vi "Initial Values-format and values-DBL.vi"() -> (1 "Values Array":dbl[](array[numeric]), 3 "Keys Array":T1)   [LabVIEW 2013]
uses:
  Typedefs/Ini file interface (DBL).ctl
  User Interface/Visualisation/Functional Imaging Viewer/Typedefs/Get-Set-Clear Control.ctl
  Global Variables/gl_UI Ctrl Refs.vi
  User Interface/Visualisation/Timelapse Viewer/Globals/gl_Time series viewer globals.vi
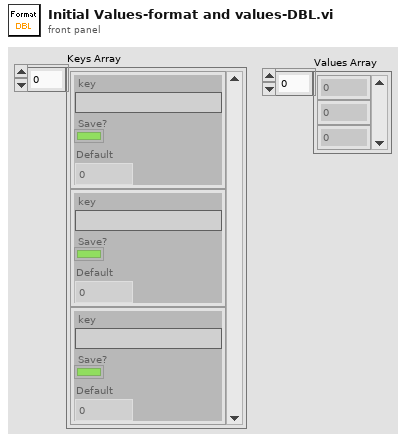
[diagram p1: front panel]
types:
  T1 = typedef "Ini file interface (DBL).ctl" = cluster{"key":string, "Save?":bool, "Default":dbl}[]
  T2 = typedef "Get-Set-Clear Control.ctl" = enum16{"Get", "Set", "Clear"}
  T3 = typedef "UI ctrl refs cluster.ctl" = cluster{"Top level VI path":path, "Top level VI ref":refnum<vi>, "User menu ref":refnum<k9>, "Sub Panel control":refnum<vi>, "Imaging Param Tab":refnum<vi>, "Occurrence-Start drivers":refnum<k4>, "Occurrence-Speed logging initialised":refnum<k4>, "Occurrence-XYZ stage initialised":refnum<k4>, "Exit button":refnum<vi>, "Status ind":refnum<vi>, "Return to Origin":refnum<vi>, "Speed Logging":refnum<vi>, "Time Lapse":refnum<vi>, "Live Imaging":refnum<vi>, "AOL Z Stack":refnum<vi>, "Motor Z Stack":refnum<vi>, "Funct Acq button":refnum<vi>, "Hard Shutter":refnum<vi>, "Virtual Shutter":refnum<vi>, "Laser Power":refnum<vi>, "AOL Mode":refnum<vi>, "Frame Size":refnum<vi>, "Field of View":refnum<vi>, "Dwell Time":refnum<vi>, "Zoom":refnum<vi>, "AOL Z":refnum<vi>, "Objective":refnum<vi>, "Axis":refnum<vi>, "Paths & Names":refnum<vi>, "Experiment folder path (ind.)":refnum<vi>, "Last State (Ind.)":refnum<vi>, "Laser wavelength ind (nm)":refnum<vi>, "Averages":refnum<vi>, "Angle (degrees)":refnum<vi>, "X centre":refnum<vi>, "Y centre":refnum<vi>, "Plane Mode":refnum<vi>, "# Planes":refnum<vi>, "Z Start":refnum<vi>, "Z Stop":refnum<vi>, "Z Step":refnum<vi>, "PMT 1":refnum<vi>, "PMT 2":refnum<vi>, "Stage XYZ Position":refnum<vi>, "Pockels@Z Start":refnum<vi>, "Pockels@Z Stop":refnum<vi>, "Obtain Z Start":refnum<vi>, "Obtain Z Stop":refnum<vi>, "Live stim.trig.period":refnum<vi>, "Live stim.trig.enable":refnum<vi>, "Funct. Acq. Pockels Modulation":refnum<vi>, "Enable Video Recording":refnum<vi>, "Video Record-Live Imaging":refnum<vi>, "Video Record-Funct acq":refnum<vi>, "AOL Z-stack Chirps Ready (ind)":refnum<vi>, "Center freq ind (nm)":refnum<vi>, "Logging queue (ind)":refnum<vi>, "Back aperture power (ind.)":refnum<vi>, "Power after objective (ind.)":refnum<vi>, "Switch user":refnum<vi>}
  T4 = typedef "AOL_Globals.ctl" = cluster{"Imaging Protocol":T5, "Number of POI":u16, "Number of Miniscans":u16, "Number of Trials":u16, "Number of Cycles ":u64, "# Averaged Frames":u16, "Laser power (%)":u8, "Pockels":dbl, "Acquisition Length (sec)":dbl, "Fill time (us)":dbl, "POI Dwell time (us)":dbl, "Miniscan Dwell time per pixel (us)":dbl, "PMT 1":dbl, "PMT 2":dbl, "Back Apperture":dbl, "Frame Size":T6, "Center Frequency":dbl, "Field of View":dbl, "DwellTime (us)":dbl, "Wavelength (nm)":dbl, "Zoom":dbl, "AOL Z":dbl, "AOL Mode":T7, "GridXY":dbl, "GridZ":dbl, "TriggerPeriod (sec)":dbl, "Number of Pixels in Miniscan":u16, "Experiment folder path":path, "X centre":dbl, "Y centre":dbl, "Angle (degrees)":dbl, "Plane Mode":T8, "Threshold":u16[], "Regenerate Chirps":bool, "Rectangle ROI length (pixels)":u16, "Rectangle ROI height (pixels)":u16, "AOD fill":u16, "Samples Wait after Trigger":u16, "StartUp Delay":i32, "Slip Cycle":u32, "Add Cycle":bool}
  T5 = typedef "Imaging Protocols enum.ctl" = enum16{"AOL Z-Stack", "Motor Z Stack", "Functional Acquisition", "Single Plane Acquisition", "Volume Acquisition", "Live Imaging", "Live Plane Imaging", "Live Volume Imaging"}
  T6 = typedef "Frame Size.ctl" = u16
  T7 = typedef "AOL modes.ctl" = enum16{"Raster", "Structural", "Pointing", "Mini Scan", "Alignment"}
  T8 = typedef "Plane Mode.ctl" = u16
  T9 = typedef "Stitch layout spec cluster.ctl" = cluster{"Timelapse image":cluster{"Image position":T10}, "Cam 1":cluster{"Image position":T10}, "Cam 2":cluster{"Image position":T10}, "Cam 3":cluster{"Image position":T10}, "Cam 4":cluster{"Image position":T10}}
  T10 = typedef "Image stitching positions.ctl" = enum16{"Top left", "Top right", "Bottom left", "Bottom right", "Not used"}
  T11 = typedef "PMT control knob.ctl" = u16
  T12 = typedef "Custom slider-horisontal.ctl" = cluster{dbl, dbl}
  T13 = typedef "Speed graph behaviour enum.ctl" = enum16{"Scrolling data", "Scrolling cursor"}
  T14 = typedef "AVI implementation enum.ctl" = enum16{"AVI1", "AVI2"}
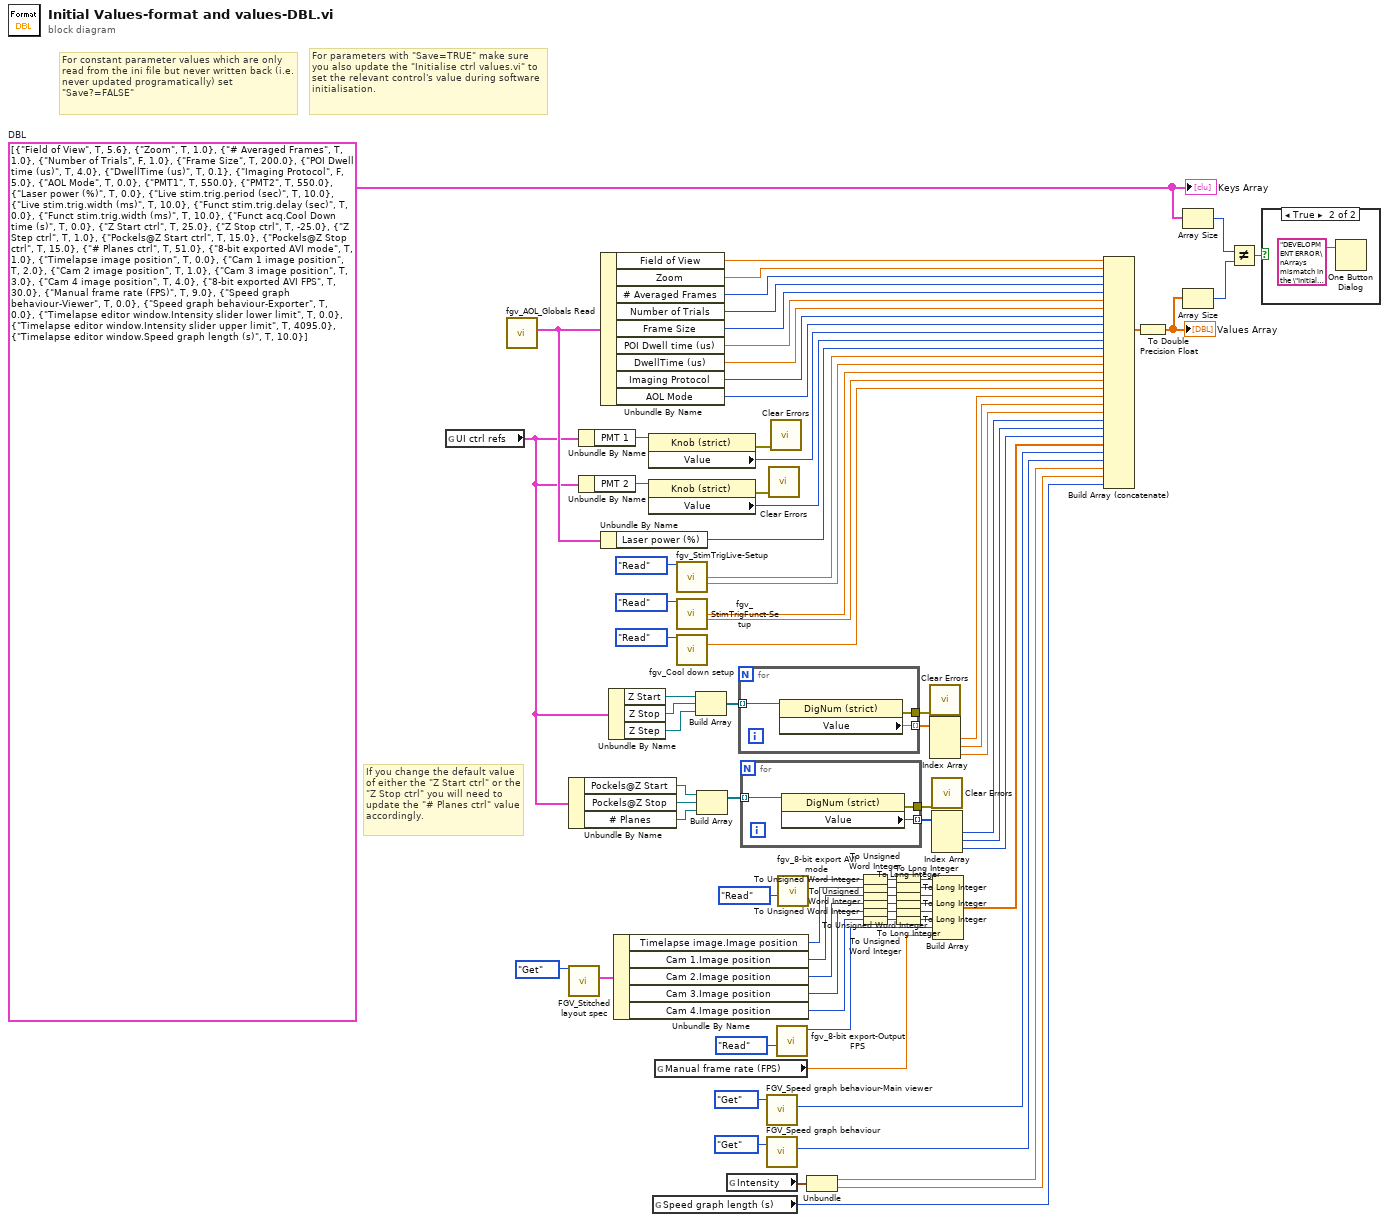
[diagram p0: block diagram]
diagram:
  w56 = T1 [{"key"="Field of View", "Save?"=TRUE, "Default"=5.6}, {"key"="Zoom", "Save?"=TRUE, "Default"=1.0}, {"key"="# Averaged Frames", "Save?"=TRUE, "Default"=1.0}, {"key"="Number of Trials", "Save?"=FALSE, "Default"=1.0}, {"key"="Frame Size", "Save?"=TRUE, "Default"=200.0}, {"key"="POI Dwell time (us)", "Save?"=TRUE, "Default"=4.0}, {"key"="DwellTime (us)", "Save?"=TRUE, "Default"=0.1}, {"key"="Imaging Protocol", "Save?"=FALSE, "Default"=5.0}, {"key"="AOL Mode", "Save?"=TRUE, "Default"=0.0}, {"key"="PMT1", "Save?"=TRUE, "Default"=550.0}, {"key"="PMT2", "Save?"=TRUE, "Default"=550.0}, {"key"="Laser power (%)", "Save?"=TRUE, "Default"=0.0}, {"key"="Live stim.trig.period (sec)", "Save?"=TRUE, "Default"=10.0}, {"key"="Live stim.trig.width (ms)", "Save?"=TRUE, "Default"=10.0}, {"key"="Funct stim.trig.delay (sec)", "Save?"=TRUE, "Default"=0.0}, {"key"="Funct stim.trig.width (ms)", "Save?"=TRUE, "Default"=10.0}, {"key"="Funct acq.Cool Down time (s)", "Save?"=TRUE, "Default"=0.0}, {"key"="Z Start ctrl", "Save?"=TRUE, "Default"=25.0}, {"key"="Z Stop ctrl", "Save?"=TRUE, "Default"=-25.0}, {"key"="Z Step ctrl", "Save?"=TRUE, "Default"=1.0}, {"key"="Pockels@Z Start ctrl", "Save?"=TRUE, "Default"=15.0}, {"key"="Pockels@Z Stop ctrl", "Save?"=TRUE, "Default"=15.0}, {"key"="# Planes ctrl", "Save?"=TRUE, "Default"=51.0}, {"key"="8-bit exported AVI mode", "Save?"=TRUE, "Default"=1.0}, {"key"="Timelapse image position", "Save?"=TRUE, "Default"=0.0}, {"key"="Cam 1 image position", "Save?"=TRUE, "Default"=2.0}, {"key"="Cam 2 image position", "Save?"=TRUE, "Default"=1.0}, {"key"="Cam 3 image position", "Save?"=TRUE, "Default"=3.0}, {"key"="Cam 4 image position", "Save?"=TRUE, "Default"=4.0}, {"key"="8-bit exported AVI FPS", "Save?"=TRUE, "Default"=30.0}, {"key"="Manual frame rate (FPS)", "Save?"=TRUE, "Default"=9.0}, {"key"="Speed graph behaviour-Viewer", "Save?"=TRUE, "Default"=0.0}, {"key"="Speed graph behaviour-Exporter", "Save?"=TRUE, "Default"=0.0}, {"key"="Timelapse editor window.Intensity slider lower limit", "Save?"=TRUE, "Default"=0.0}, {"key"="Timelapse editor window.Intensity slider upper limit", "Save?"=TRUE, "Default"=4095.0}, {"key"="Timelapse editor window.Speed graph length (s)", "Save?"=TRUE, "Default"=10.0}]  # DBL
  # "If you change the default value of either the \"Z Start ctrl\" or the \"Z Stop ctrl\" you will need to update the \"# Planes ctrl\" value accordingly."
  # "For parameters with \"Save=TRUE\" make sure you also update the \"Initialise ctrl values.vi\" to set the relevant control's value during software initialisation."
  # "For constant parameter values which are only read from the ini file but never written back (i.e. never updated programatically) set \"Save?=FALSE\""
  n1 = global read "gl_UI Ctrl Refs.vi" "UI ctrl refs"() -> (w45:T3)
  n2 = call "fgv_AOL_Globals Read.vi"() -> ("AOL_Globals"=w70:T4)  [unwired: 9 in, 2 out]
  n3 = Unbundle By Name(w45) -> ("Pockels@Z Start"=w46:refnum<vi>, "Pockels@Z Stop"=w47:refnum<vi>, "# Planes"=w37:refnum<vi>)
  n4 = call "FGV_Stitched layout spec.vi"("Function"=Get-Set-Clear_Control."Get") -> ("Stitch layout spec"=w31:T9)  [unwired: 9 in, 1 out]
  n5 = Unbundle By Name(w45) -> ("PMT 1"=w73:refnum<vi>)
  n6 = Unbundle By Name(w45) -> ("PMT 2"=w72:refnum<vi>)
  n7 = Unbundle By Name(w70) -> ("Field of View"=w59:dbl, "Zoom"=w60:dbl, "# Averaged Frames"=w62:u16, "Number of Trials"=w61:u16, "Frame Size"=w63:T6, "POI Dwell time (us)"=w64:dbl, "DwellTime (us)"=w65:dbl, "Imaging Protocol"=w66:T5, "AOL Mode"=w67:T7)
  n8 = Unbundle By Name(w70) -> ("Laser power (%)"=w71:u8)
  n9 = Unbundle By Name(w45) -> ("Z Start"=w52:refnum<vi>, "Z Stop"=w50:refnum<vi>, "Z Step"=w49:refnum<vi>)
  n10 = Unbundle By Name(w31) -> ("Timelapse image.Image position"=w30:T10, "Cam 1.Image position"=w29:T10, "Cam 2.Image position"=w28:T10, "Cam 3.Image position"=w27:T10, "Cam 4.Image position"=w26:T10)
  n11 = property class="Knob (strict)"(reference=w73) -> (error out=w74:errorcluster, "Value"=w68:T11)  [unwired: 1 in, 1 out]
  n12 = property class="Knob (strict)"(reference=w72) -> (error out=w75:errorcluster, "Value"=w69:T11)  [unwired: 1 in, 1 out]
  n13 = global read "gl_Time series viewer globals.vi" "Speed graph length (s)"() -> (w1:i32)
  n14 = global read "gl_Time series viewer globals.vi" "Manual frame rate (FPS)"() -> (w12:dbl)
  n15 = call "fgv_StimTrigLive-Setup.vi"("Function"=enum16{"Intialize", "Write", "Read", "Clear"}."Read") -> ("Live stim.trig.period (sec)"=w78:dbl, "Live stim.trig.width (ms)"=w79:dbl)  [unwired: 11 in, 2 out]
  n16 = call "fgv_StimTrigFunct-Setup.vi"("Function"=enum16{"Intialize", "Write", "Read", "Clear"}."Read") -> ("Funct stim.trig.delay (sec)"=w80:dbl, "Funct stim.trig.width (ms)"=w81:dbl)  [unwired: 11 in, 2 out]
  n17 = call "fgv_Cool down setup.vi"("Function"=enum16{"Intialize", "Write", "Read", "Clear"}."Read") -> ("Cool-down time (s)"=w83:dbl)  [unwired: 12 in, 2 out]
  n18 = Build Array(w52, w50, w49) -> (w51:refnum<vi>[])
  n19 = Build Array(w46, w47, w37) -> (w43:refnum<vi>[])
  n20 = global read "gl_Time series viewer globals.vi" "Intensity"() -> (w4:T12)
  n21 = for {
    tunnel: w51 -> [w86] mode=indexing
    tunnel: [w85] -> w48 mode=indexing
    tunnel: [w84] -> w10
    n22 = property class="DigNum (strict)"(reference=w86) -> (error out=w84:errorcluster, "Value"=w85:dbl)  [unwired: 1 in, 1 out]
  }
  n23 = for {
    tunnel: w43 -> [w89] mode=indexing
    tunnel: [w88] -> w44 mode=indexing
    tunnel: [w87] -> w9
    n24 = property class="DigNum (strict)"(reference=w89) -> (error out=w87:errorcluster, "Value"=w88:u16)  [unwired: 1 in, 1 out]
  }
  n25 = call "FGV_Speed graph behaviour-Main viewer.vi"("Function"=Get-Set-Clear_Control."Get") -> ("Speed graph behaviour"=w6:T13)  [unwired: 9 in, 1 out]
  n26 = call "FGV_Speed graph behaviour.vi"("Function"=Get-Set-Clear_Control."Get") -> ("Speed graph behaviour"=w5:T13)  [unwired: 9 in, 1 out]
  n27 = call <vilib>:"Clear Errors.vi"("error in (no error)"=w75) -> ()  [unwired: 6 in, 1 out]
  n28 = call <vilib>:"Clear Errors.vi"("error in (no error)"=w74) -> ()  [unwired: 6 in, 1 out]
  n29 = call "fgv_8-bit export-Output FPS.vi"("Function"=enum16{"Intialize", "Write", "Read", "Clear"}."Read") -> ("Frames Per Second"=w35:u32)  [unwired: 9 in, 1 out]
  n30 = call "fgv_8-bit export AVI mode.vi"("Function"=enum16{"Intialize", "Write", "Read", "Clear"}."Read") -> ("AVI mode"=w33:T14)  [unwired: 9 in, 1 out]
  n31 = Unbundle(w4) -> (w3:dbl, w2:dbl)
  n32 = To Unsigned Word Integer(number=w33) -> (unsigned 16bit integer=w19:u16)
  n33 = To Unsigned Word Integer(number=w30) -> (unsigned 16bit integer=w18:u16)
  n34 = To Unsigned Word Integer(number=w29) -> (unsigned 16bit integer=w17:u16)
  n35 = To Unsigned Word Integer(number=w28) -> (unsigned 16bit integer=w16:u16)
  n36 = To Unsigned Word Integer(number=w27) -> (unsigned 16bit integer=w15:u16)
  n37 = To Unsigned Word Integer(number=w26) -> (unsigned 16bit integer=w14:u16)
  n38 = To Long Integer(number=w19) -> (32bit integer=w24:i32)
  n39 = To Long Integer(number=w18) -> (32bit integer=w25:i32)
  n40 = To Long Integer(number=w17) -> (32bit integer=w23:i32)
  n41 = To Long Integer(number=w16) -> (32bit integer=w22:i32)
  n42 = To Long Integer(number=w15) -> (32bit integer=w21:i32)
  n43 = To Long Integer(number=w14) -> (32bit integer=w20:i32)
  n44 = call <vilib>:"Clear Errors.vi"("error in (no error)"=w10) -> ()  [unwired: 6 in, 1 out]
  n45 = Index Array(array=w48) -> (element #1=w42:dbl, element #2=w41:dbl, element #3=w40:dbl)  [unwired: 3 in]
  n46 = call <vilib>:"Clear Errors.vi"("error in (no error)"=w9) -> ()  [unwired: 6 in, 1 out]
  n47 = Index Array(array=w44) -> (element #1=w39:u16, element #2=w38:u16, element #3=w36:u16)  [unwired: 3 in]
  n48 = Build Array(w24, w25, w23, w22, w21, w20, w35, w12) -> (w11:dbl[])
  n49 = Build Array (concatenate)(w59, w60, w62, w61, w63, w64, w65, w66, w67, w68, w69, w71, w78, w79, w80, w81, w83, w42, w41, w40, w39, w38, w36, w11, w6, w5, w3, w2, w1) -> (w58:dbl[])
  n50 = To Double Precision Float(number=w58) -> (double precision float=w57:dbl[])
  "Values Array" <- w57
  n51 = Array Size(array=w56) -> (size(s)=w55:i32)
  n52 = Array Size(array=w57) -> (size(s)=w54:i32)
  n53 = Not Equal?(x=w55, y=w54) -> (x != y?=w53:bool)
  n54 = case shown="True" w53 {
    frame False {
    }
    frame True {
      n55 = One Button Dialog(message="DEVELOPMENT ERROR\nArrays mismatch in the \"Initial Values-format and values-DBL.vi\"") -> ()  [unwired: 1 in, 1 out]
    }
  }
  "Keys Array" <- w56
